vi "Initialize Hardware References.vi"(8 "error in (no error)":errorcluster, 11 "Hardware Resources in":T1={"Test Setting"={"Test_Num"=0, "Test_ID"=0, "Proc_ID"=0, "Max Force"=0.0, "User"="", "SN"="", "Date"=""}, "Measurements"=[[""]], "LOG REF"=refnum, "Report Template"=path "", "Save Report path"=path "", "Data File Path"=path "", "Popup Dialog"=FALSE}) -> (0 "error out":errorcluster, 2 "report out":refnum<class "NI_report.lvclass">, 3 "Hardware Resources out":T1)   [LabVIEW 2020, in "Report.lvlib"]
doc: "Initialize the hardware references."
uses:
  Report.lvlib
  REP Configuration.ctl
  Test Setting.ctl
  <vilib>/Utility/NIReport.llb/NI_report.lvclass
  <vilib>/Utility/NIReport.llb/Report Type.ctl
  <vilib>/Utility/NIReport.llb/NI_ReportGenerationCore.lvlib
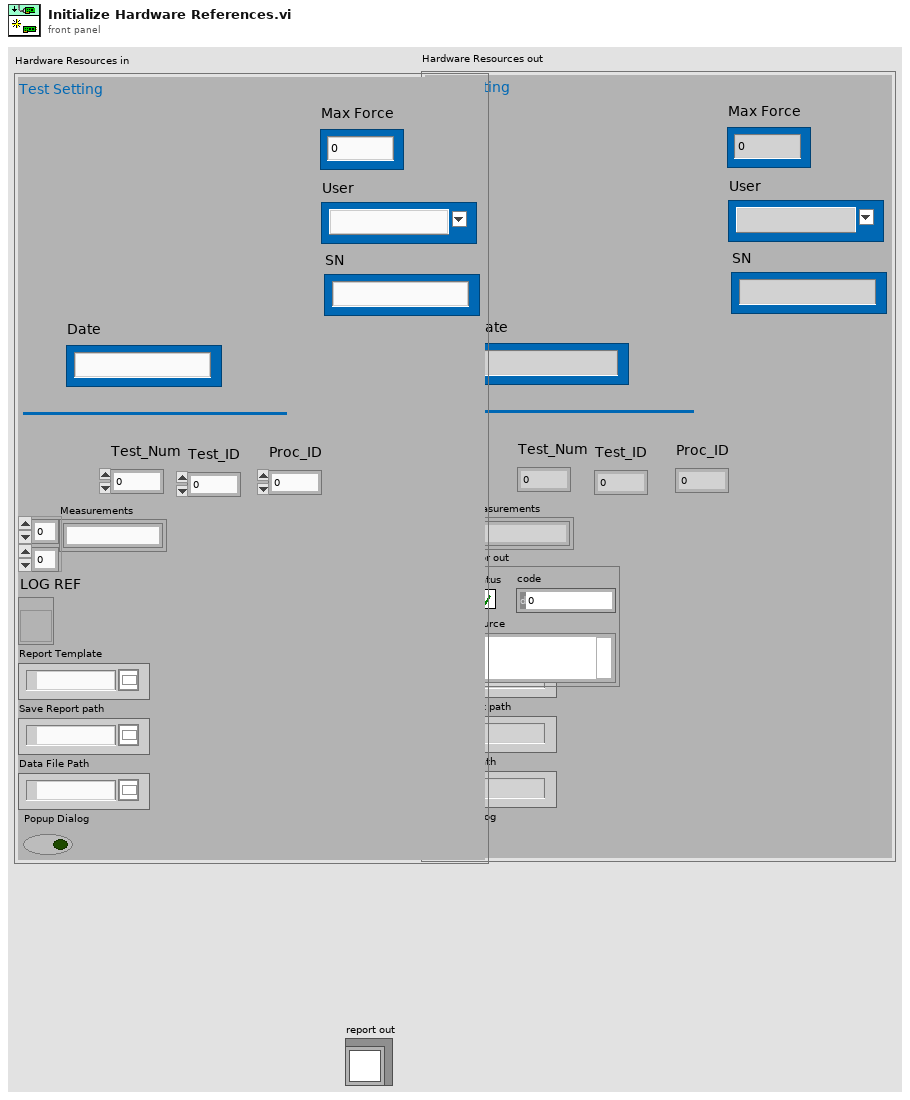
[diagram p1: front panel]
types:
  T1 = typedef "Report.lvlib/REP Configuration.ctl" = cluster{"Test Setting":T2, "Measurements":string[][], "LOG REF":refnum<vi>, "Report Template":path, "Save Report path":path, "Data File Path":path, "Popup Dialog":bool}
  T2 = typedef "Report.lvlib/Test Setting.ctl" = cluster{"Test_Num":i32, "Test_ID":i32, "Proc_ID":i32, "Max Force":dbl, "User":string, "SN":string, "Date":string}
  T3 = typedef "NI_ReportGenerationCore.lvlib/Report Type.ctl" = enum16{"HTML", "Word", "Excel"}
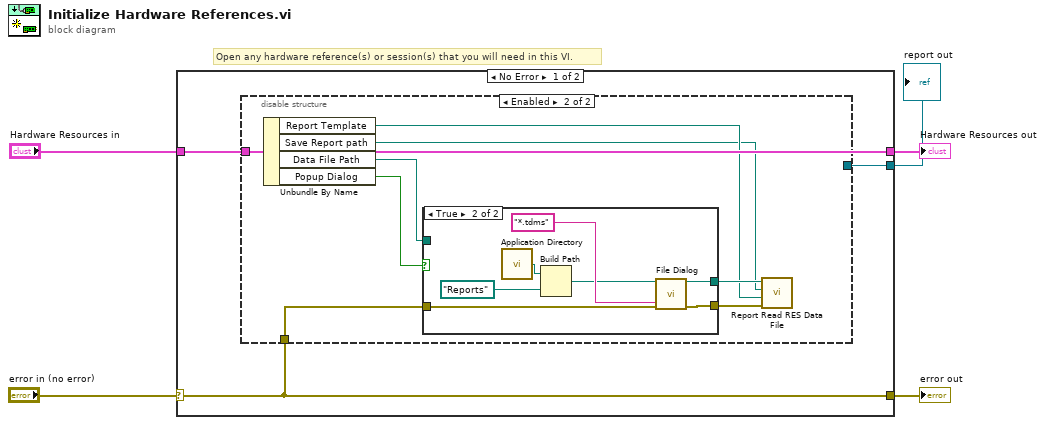
[diagram p0: block diagram]
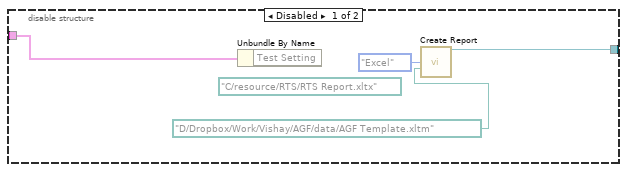
[diagram p2: hidden frame]
diagram:
  # "Open any hardware reference(s) or session(s) that you will need in this VI."
  n1 = case shown="No Error" "error in (no error)" {
    selector: "error in (no error)" -> [w6 w30]
    tunnel: [w6 w30] -> w4
    tunnel: "Hardware Resources in" -> [w7 w31]
    tunnel: [w7 w31] -> w2
    tunnel: [w8 _] -> w1
    frame No Error {
      n2 = disable-structure shown="Enabled" {
        disable-tunnel: [w12 _] -> w8
        disable-tunnel: w7 -> [w9 w16]
        disable-tunnel: w6 -> [_ w15]
        frame Disabled {
          (unwired) path "C:/resource/RTS/RTS Report.xltx" ("template (empty)")
          n3 = Unbundle By Name(w9) -> ()  [unwired: 1 out]
          n4 = call <vilib>:"Create Report.vi"("report type"=Report_Type."Excel", "template (empty)"=path "D:/Dropbox/Work/Vishay/AGF/data/AGF Template.xltm") -> ("report out"=w12:refnum<class "NI_report.lvclass">)  [unwired: 12 in, 1 out]
        }
        frame Enabled {
          n5 = Unbundle By Name(w16) -> ("Report Template"=w18:path, "Save Report path"=w17:path, "Data File Path"=w13:path, "Popup Dialog"=w14:bool)
          n6 = case shown="True" w14 {
            tunnel: [w22 w25] -> w20
            tunnel: [w21 w24] -> w19
            tunnel: w15 -> [w21 w23]
            tunnel: w13 -> [w22 _]
            frame False {
            }
            frame True {
              n7 = call <vilib>:"Application Directory.vi"() -> ("Application Directory"=w29:path)
              n8 = Build Path(base path=w29, name or relative path=path "Reports") -> (appended path=w26:path)
              n9 = call "File Dialog"("start path"=w26, "error in"=w23, "pattern (all files)"="*.tdms" ("format string")) -> ("selected path"=w25:path, "error out"=w24:errorcluster)  [unwired: 9 in, 2 out]
            }
          }
          n10 = call "Report Read RES Data File.vi"("error in (no error)"=w19, "template (empty)"=w18, "Save Report Path"=w17, "RED Data File"=w20) -> ()  [unwired: 7 in, 1 out]
        }
      }
    }
    frame Error {
    }
  }
  "Hardware Resources out" <- w2
  "error out" <- w4
  "report out" <- w1
